vi "PlotDrag-Mouse Down.vi"(0 "XYGraph ref":refnum<vi>, 7 "Coords":T2, 11 "error in (no error)":errorcluster) -> (4 "Drag State":T1, 8 "Selection":i32, 15 "error out":errorcluster)   [LabVIEW 2020]
uses:
  <vilib>/Utility/miscctls.llb/LVPoint32TypeDef.ctl
  PlotDrag-State.ctl
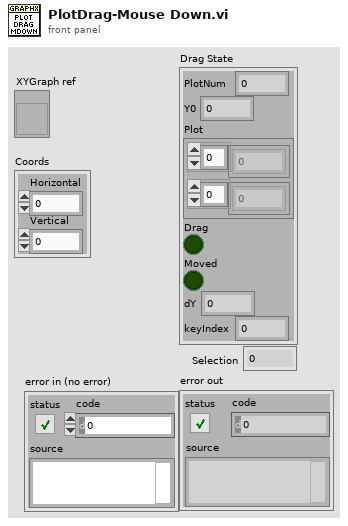
[diagram p1: front panel]
types:
  T1 = typedef "PlotDrag-State.ctl" = cluster{"PlotNum":i32, "Y0":dbl, "Plot":cluster{dbl[], dbl[]}, "Drag":bool, "Moved":bool, "dY":dbl, "keyIndex":i32}
  T2 = typedef "LVPoint32TypeDef.ctl" = cluster{"Horizontal":i32, "Vertical":i32}
  T3 = cluster{"PlotNum":i32, "Y":dbl, cluster{dbl[], dbl[]}, bool, bool, dbl, i32}
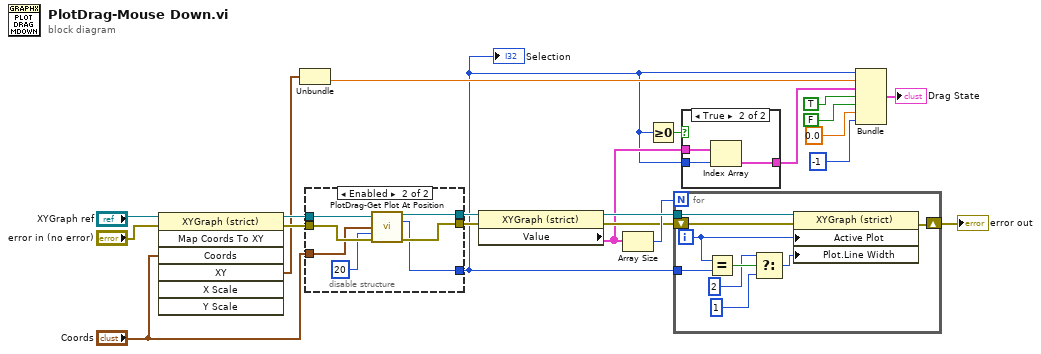
[diagram p0: block diagram]
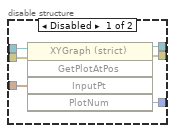
[diagram p2: hidden frame]
diagram:
  n1 = invoke class="XYGraph (strict)" method="Map Coords To XY"(reference="XYGraph ref", error in="error in (no error)", "Coords"="Coords") -> (reference out=w17:refnum<vi>, error out=w16:errorcluster, "XY"=w4:cluster{"X":dbl, "Y":dbl})  [unwired: 4 in, 4 out]
  n2 = Unbundle(w4) -> ("Y"=w9:dbl)  [unwired: 1 out]
  n3 = disable-structure shown="Enabled" {
    disable-tunnel: "Coords" -> [w28 w30]
    disable-tunnel: w17 -> [w27 w35]
    disable-tunnel: w16 -> [w26 w34]
    disable-tunnel: [w25 w33] -> w15
    disable-tunnel: [w24 w32] -> w14
    disable-tunnel: [w23 w31] -> w5
    frame Disabled {
      n4 = invoke class="XYGraph (strict)" method="GetPlotAtPos"(reference=w27, error in=w26, "InputPt"=w28) -> (reference out=w25:refnum<vi>, error out=w24:errorcluster, "PlotNum"=w23:i32)  [unwired: 2 in, 2 out]
    }
    frame Enabled {
      n5 = call "PlotDrag-Get Plot At Position.vi"("XYGraph in"=w35, "Coords"=w30, "Threshold"=20, "error in (no error)"=w34) -> ("XYGraph out"=w33:refnum<vi>, "PlotNum"=w31:i32, "error out"=w32:errorcluster)  [unwired: 8 in, 1 out]
    }
  }
  "Selection" <- w5
  n6 = property class="XYGraph (strict)"(reference=w15, error in=w14) -> (reference out=w21:refnum<vi>, error out=w13:errorcluster, "Value"=w10:cluster{dbl[], dbl[]}[])
  n7 = Array Size(array=w10) -> (size(s)=w20:i32)
  n8 = Greater Or Equal To 0?(x=w5) -> (x >= 0?=w11:bool)
  n9 = for {
    N: w20 -> [_]
    tunnel: w21 -> [w44]
    tunnel: w5 -> [w43]
    shift-right: [w36] -> w12
    shift-left: w13 -> [w37]
    i -> [w42]
    n10 = Equal?(x=w42, y=w43) -> (x = y?=w41:bool)
    n11 = Select(t=2, s=w41, f=1) -> (s? t:f=w38:i32)
    n12 = property class="XYGraph (strict)"(reference=w44, error in=w37, "Active Plot"=w42, "Plot.Line Width"=w38) -> (error out=w36:errorcluster)  [unwired: 1 out]
  }
  "error out" <- w12
  n13 = case shown="True" w11 {
    tunnel: w10 -> [_ w47]
    tunnel: w5 -> [_ w46]
    tunnel: [_ w45] -> w8
    frame False {
    }
    frame True {
      n14 = Index Array(array=w47, index=w46) -> (element=w45:cluster{dbl[], dbl[]})
    }
  }
  n15 = Bundle("PlotNum"=w5, "Y"=w9, w8, TRUE, FALSE, 0.0, -1) -> (→"Drag State":T3)  [unwired: 1 in]
